vi "FindNumbersNext.vi"(9 "Cluster":cluster{"Numeric":i32, "Numeric":i32}, 10 "Numeric":u8, 11 "Map":u8[][](array[numeric])) -> (3 "Array":cluster{"Numeric":i32, "Numeric":i32}[](array[cluster]))   [LabVIEW 2023, in "2024_10.lvclass"]
uses:
  2024_10.lvclass
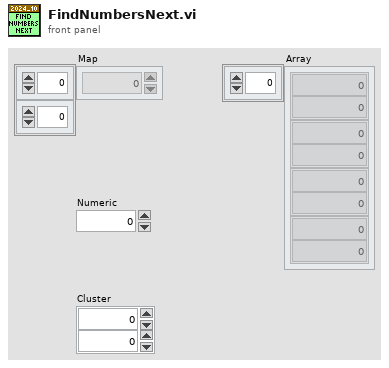
[diagram p1: front panel]
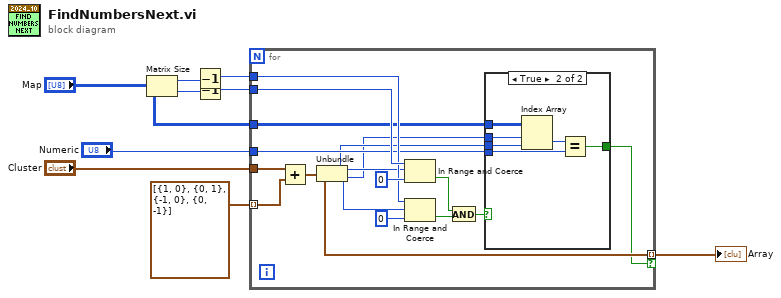
[diagram p0: block diagram]
diagram:
  n1 = Matrix Size(0:"Map") -> (1:w3:i32, 2:w4:i32)
  n2 = Decrement(x=w3) -> (x-1=w6:i32)
  n3 = Decrement(x=w4) -> (x-1=w5:i32)
  n4 = for {
    tunnel: "Cluster" -> [w24]
    tunnel: cluster{i32, i32}[] [{1, 0}, {0, 1}, {-1, 0}, {0, -1}] ("y") -> [w23] mode=indexing
    tunnel: w5 -> [w21]
    tunnel: w6 -> [w19]
    tunnel: "Map" -> [w15]
    tunnel: "Numeric" -> [w14]
    tunnel: [w13] -> w9 mode=indexing if=w12
    n5 = Add(x=w24, y=w23) -> (x+y=w13:cluster{i32, i32})
    n6 = Unbundle(w13) -> (w11:i32, w10:i32)
    n7 = In Range and Coerce(upper limit=w21, x=w11, lower limit=0) -> (In Range?=w17:bool)  [unwired: 1 out]
    n8 = In Range and Coerce(upper limit=w19, x=w10, lower limit=0) -> (In Range?=w18:bool)  [unwired: 1 out]
    n9 = And(x=w17, y=w18) -> (x .and. y?=w16:bool)
    n10 = case shown="True" w16 {
      tunnel: w15 -> [_ w30]
      tunnel: w14 -> [_ w28]
      tunnel: [_ w27] -> w12
      tunnel: w11 -> [_ w26]
      tunnel: w10 -> [_ w25]
      frame False {
      }
      frame True {
        n11 = Index Array(array=w30, index (row)=w25, index (col)=w26) -> (element=w29:u8)
        n12 = Equal?(x=w29, y=w28) -> (x = y?=w27:bool)
      }
    }
  }
  "Array" <- w9
